vi "Test Confluence VIDoc.vi"() -> ()   [LabVIEW 2023]
uses:
  <vilib>/DMC/VIDoc/Framework/UI Interaction/Progress Bar UI/Progress Bar UI.lvclass
  C:/Program Files/National Instruments/LabVIEW 2023/vi.lib/DMC/VIDoc/Framework/UI Interaction/Interface/UI Interaction.lvclass
  <vilib>/DMC/VIDoc/Printers/Confluence/Confluence Printer/VIDoc Printer - Confluence.lvclass
  <vilib>/DMC/VIDoc/Framework/Parsing/Documentation Parser/VIDoc Parser.lvclass
panel:
  in  "Top Page ID":string
  in  "Git History?":bool
  in  "Source Root":path
  in  "VIDoc json Settings Path":path
  out "Group":string
  out "Section":string
  out "error out":errorcluster {"code" format="Error %.0f"}
  out "Message":string
  out "Progress Bar":i32(slide) max=28 scale=0.0..7.0
  in  "Abort":bool
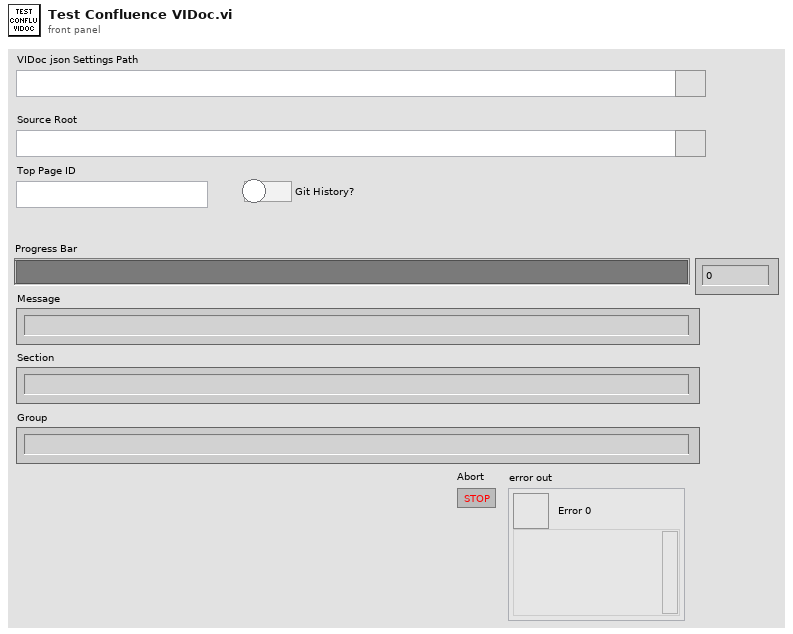
[diagram p1: front panel]
types:
  T1 = cluster{"Progress Max":refnum<user-event>, "Progress Value":refnum<user-event>, "Message":refnum<user-event>, "Stopped":refnum<user-event>, "Section":refnum<user-event>, "Group":refnum<user-event>}
  T2 = typedef "VIDoc Printer - Confluence.lvlib/VIDoc Printer - Confluence.lvclass/File Change Map.ctl" = map{string, cluster{"Timestamp":timestamp, "Commit Hash":string, "Author Name":string, "Branch":string, "Commit Hash URL":string}}
  T3 = typedef "VIDoc Parsing.lvlib/Full Documentation Info.ctl" = cluster{"Projects":refnum<class "Project Documentation.lvclass">[], "Interfaces":refnum<class "Interface Documenation.lvclass">[], "Classes":refnum<class "Class Documentation.lvclass">[], "Libraries":refnum<class "Library Documentation.lvclass">[], "VI Members":refnum<class "GUI Documentation.lvclass">[], "Controls":refnum<class "GUI Documentation.lvclass">[], "LLBs":refnum<class "LLB Documentation.lvclass">[], "Bookmarked Map":map{string, refnum<class "GUI Documentation.lvclass">[]}}
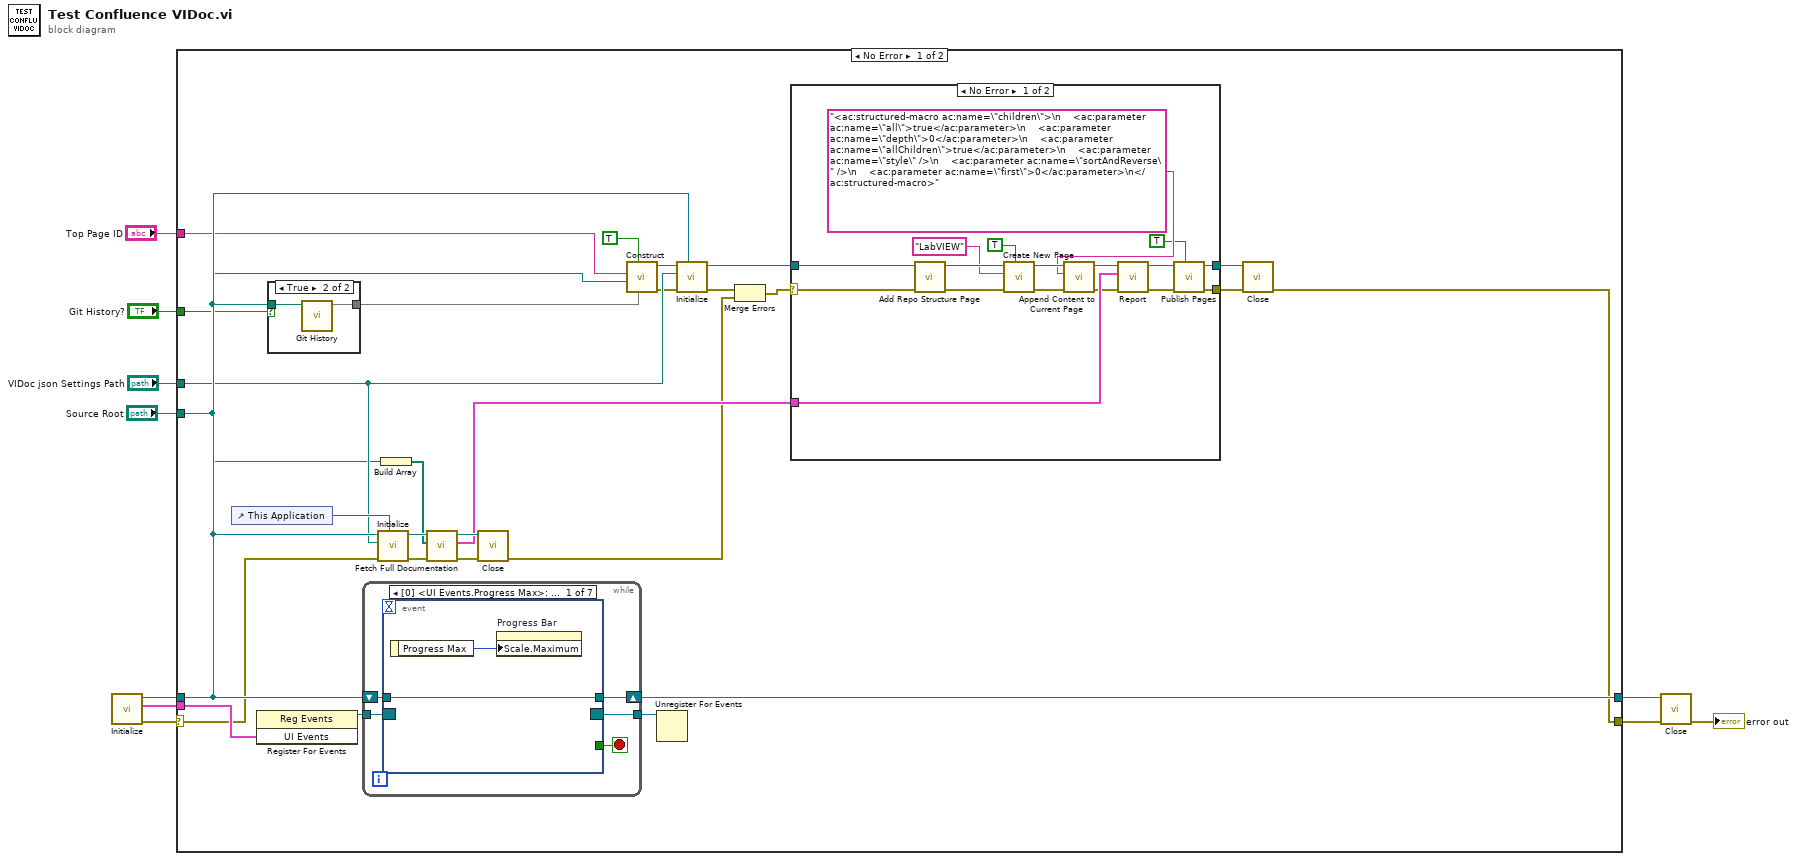
[diagram p0: block diagram]
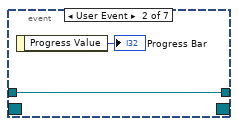
[diagram p3: hidden frame]
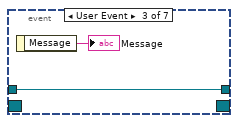
[diagram p4: hidden frame]
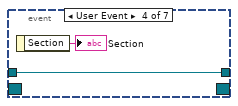
[diagram p5: hidden frame]
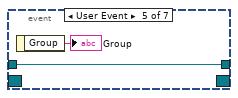
[diagram p6: hidden frame]
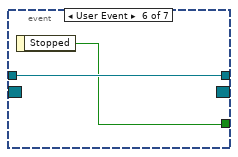
[diagram p7: hidden frame]
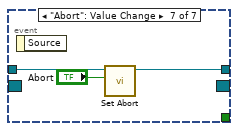
[diagram p8: hidden frame]
diagram:
  n1 = call <vilib>:"Initialize.vi"() -> ("error out"=w7:errorcluster, "UI Events"=w10:T1, "Progress Bar UI Out"=w8:refnum<class "Progress Bar UI.lvclass">)  [unwired: 9 in]
  n2 = case shown="No Error" w7 {
    selector: w7 -> [w25 w81]
    tunnel: w10 -> [w38 _]
    tunnel: [w36 w80] -> w9
    tunnel: w8 -> [w35 w80]
    tunnel: [w30 w81] -> w6
    tunnel: "VIDoc json Settings Path" -> [w24 _]
    tunnel: "Source Root" -> [w23 _]
    tunnel: "Git History?" -> [w22 _]
    tunnel: "Top Page ID" -> [w21 _]
    frame No Error {
      n3 = control-ref of="This Application"() -> (w27:refnum<vi>)
      n4 = register-events(w38) -> (reference out=w37:refnum<event-registration>)  [unwired: 2 in, 1 out]
      n5 = case shown="True" w22 {
        tunnel: [_ w79] -> w26
        tunnel: w23 -> [_ w78]
        frame False {
        }
        frame True {
          n6 = call "Git History.vi"("Working Directory"=w78) -> ("File Change Map"=w79:T2)  [unwired: 9 in, 1 out]
        }
      }
      n7 = while {
        tunnel: w37 -> [w62]
        shift-right: [w60] -> w36
        shift-left: w35 -> [w61]
        tunnel: [w58] -> w20
        stop <- w59 stop-if-true
        n8 = event shown="[0] <UI Events.Progress Max>: User Event" {
          selector: w62 -> [_ _ _ _ _ _ _]
          dyn-events: [_ _ _ _ _ _ _] -> w58
          timeout: _ -> [_ _ _ _ _ _ _]
          tunnel: w61 -> [w64 w66 w68 w70 w72 w74 w76]
          tunnel: [w64 w66 w68 w70 w72 w74 w77] -> w60
          tunnel: [_ _ _ _ _ w73 _] -> w59
          event User Event {
            n9 = event-data() -> ("Progress Max"=w63:i32)  [unwired: 1 in]
            n10 = property on="Progress Bar" class="Slide (strict)"("Scale.Maximum"=w63) -> ()  [unwired: 2 in, 2 out]
          }
          event User Event {
            n11 = event-data() -> ("Progress Value"=→"Progress Bar":i32)  [unwired: 1 in]
          }
          event User Event {
            n12 = event-data() -> ("Message"=→"Message":string)  [unwired: 1 in]
          }
          event User Event {
            n13 = event-data() -> ("Section"=→"Section":string)  [unwired: 1 in]
          }
          event User Event {
            n14 = event-data() -> ("Group"=→"Group":string)  [unwired: 1 in]
          }
          event User Event {
            n15 = event-data() -> ("Stopped"=w73:bool)  [unwired: 1 in]
          }
          event "Abort": Value Change {
            n16 = event-data() -> ()  [unwired: 1 in, 1 out]
            n17 = call <vilib>:"Set Abort.vi"("Abort?"="Abort", "Progress Bar UI In"=w76) -> ("Progress Bar UI Out"=w77:refnum<class "Progress Bar UI.lvclass">)  [unwired: 8 in, 1 out]
          }
        }
      }
      n18 = call <vilib>:"Initialize.vi"("App Reference (This Application)"=w27, "error in (no error)"=w25, "Settings Path"=w24, "UI Interaction"=w35) -> ("error out"=w34:errorcluster, "VIDoc Parser Out"=w33:refnum<class "VIDoc Parser.lvclass">)  [unwired: 6 in]
      n19 = Build Array(w23) -> (w28:path[])
      n20 = call <vilib>:"Fetch Full Documentation.vi"("error in (no error)"=w34, "File Paths"=w28, "VIDoc Parser In"=w33) -> ("error out"=w31:errorcluster, "Full Documentation"=w29:T3, "VIDoc Parser Out"=w32:refnum<class "VIDoc Parser.lvclass">)  [unwired: 6 in]
      n21 = call <vilib>:"Close.vi"("error in (no error)"=w31, "VIDoc Parser In"=w32) -> ("error out"=w11:errorcluster)  [unwired: 9 in]
      n22 = call <vilib>:"Construct.vi"("File Change Map"=w26, "Bulk Attachments? (T)"=TRUE, "Working Directory"=w23, "Top Page ID"=w21) -> ("error out"=w19:errorcluster, "VIDoc Printer - Confluence Out"=w18:refnum<class "VIDoc Printer - Confluence.lvclass">)  [unwired: 6 in]
      n23 = Unregister For Events(event registration refnum=w20) -> ()  [unwired: 1 in, 1 out]
      n24 = call-dynamic <vilib>:"Initialize.vi"("UI Interaction"=w35, "error in (no error)"=w19, "Settings Path"=w24, "VIDoc Printer - Confluence In"=w18) -> ("error out"=w17:errorcluster, "VIDoc Printer - Confluence Out"=w16:refnum<class "VIDoc Printer - Confluence.lvclass">)  [unwired: 6 in]
      n25 = Merge Errors(w17, w11) -> (w12:errorcluster)
      n26 = case shown="No Error" w12 {
        selector: w12 -> [w54 w56]
        tunnel: w29 -> [w55 _]
        tunnel: w16 -> [w53 w57]
        tunnel: [w52 w56] -> w14
        tunnel: [w51 w57] -> w13
        frame No Error {
          n27 = call <vilib>:"Add Repo Structure Page.vi"("error in (no error)"=w54, "VIDoc Printer - Confluence In"=w53) -> ("error out"=w48:errorcluster, "VIDoc Printer - Confluence Out"=w47:refnum<class "VIDoc Printer - Confluence.lvclass">)  [unwired: 8 in]
          n28 = call <vilib>:"Create New Page.vi"("Update Current Page (F)"=TRUE, "error in (no error)"=w48, "Name"="LabVIEW", "VIDoc Printer - Confluence In"=w47) -> ("error out"=w42:errorcluster, "VIDoc Printer - Confluence Out"=w44:refnum<class "VIDoc Printer - Confluence.lvclass">)  [unwired: 4 in, 2 out]
          n29 = call <vilib>:"Append Content to Current Page.vi"("error in (no error)"=w42, "Content"="<ac:structured-macro ac:name=\"children\">\n    <ac:parameter ac:name=\"all\">true</ac:parameter>\n    <ac:parameter ac:name=\"depth\">0</ac:parameter>\n    <ac:parameter ac:name=\"allChildren\">true</ac:parameter>\n    <ac:parameter ac:name=\"style\" />\n    <ac:parameter ac:name=\"sortAndReverse\" />\n    <ac:parameter ac:name=\"first\">0</ac:parameter>\n</ac:structured-macro>", "VIDoc Printer - Confluence In"=w44) -> ("error out"=w41:errorcluster, "VIDoc Printer - Confluence Out"=w43:refnum<class "VIDoc Printer - Confluence.lvclass">)  [unwired: 7 in]
          n30 = call-dynamic "Report.vi"("error in (no error)"=w41, "Full Documentation"=w55, "VIDoc Printer In"=w43) -> ("error out"=w50:errorcluster, "VIDoc Printer Out"=w49:refnum<class "VIDoc Printer - Confluence.lvclass">)  [unwired: 7 in]
          n31 = call <vilib>:"Publish Pages.vi"("Parallel?"=TRUE, "error in (no error)"=w50, "VIDoc Printer - Confluence In"=w49) -> ("error out"=w52:errorcluster, "VIDoc Printer - Confluence Out"=w51:refnum<class "VIDoc Printer - Confluence.lvclass">)  [unwired: 7 in]
        }
        frame Error {
        }
      }
      n32 = call-dynamic <vilib>:"Close.vi"("error in (no error)"=w14, "VIDoc Printer - Confluence In"=w13) -> ("error out"=w30:errorcluster)  [unwired: 9 in]
    }
    frame Error {
    }
  }
  n33 = call <vilib>:"Close.vi"("error in (no error)"=w6, "Progress Bar UI In"=w9) -> ("error out"=→"error out":errorcluster)  [unwired: 9 in]
